vi "ChangeMotionParams.vi"(4 "newTrqGlobal":i32=4, 6 "newTrackingLimit":u32=100, 7 "newVelLimit":i32=2000, 8 "error in (no error)":errorcluster, 9 "newJrkLimit":i32=3, 10 "newAccelLimit":dbl format="%#_13g", 11 "Axis in":refnum<class "Axis.lvclass">) -> (0 "error out":errorcluster, 3 "Axis out":refnum<class "Axis.lvclass">)   [LabVIEW 2020, in "Axis.lvclass"]
uses:
  Axis.lvclass
  Axis.lvclass/Axis.ctl
  C:/Users/Jonathan/Documents/Clearpath SDK/CSharp Examples/CLRWrapper/x64/Debug/CLRWrapper.dll
  CSharp Examples/CLRWrapper/x64/Debug/CLRWrapper.dll
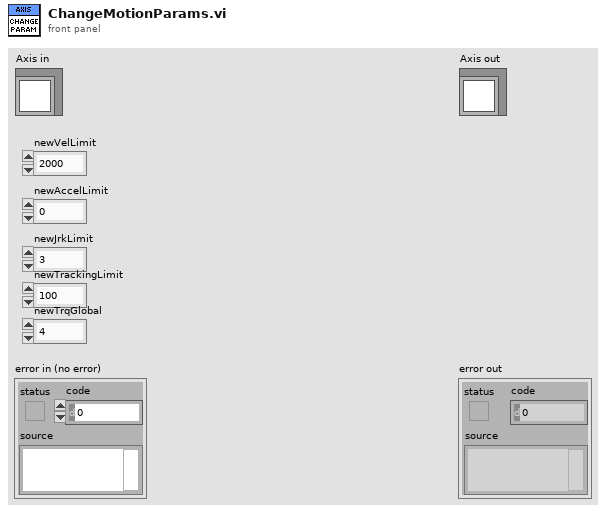
[diagram p1: front panel]
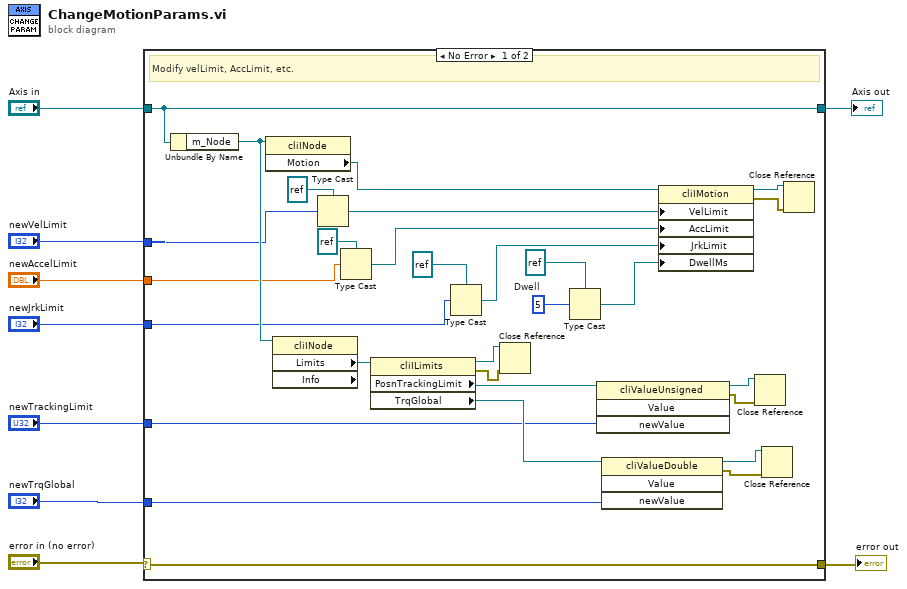
[diagram p0: block diagram]
diagram:
  n1 = case shown="No Error" "error in (no error)" {
    selector: "error in (no error)" -> [w38 w39]
    tunnel: [w38 w39] -> w4
    tunnel: "newVelLimit" -> [w36 _]
    tunnel: "newJrkLimit" -> [w35 _]
    tunnel: "Axis in" -> [w34 _]
    tunnel: [w34 _] -> w6
    tunnel: "newAccelLimit" -> [w20 _]
    tunnel: "newTrackingLimit" -> [w19 _]
    tunnel: "newTrqGlobal" -> [w18 _]
    frame No Error {
      w21 = 5  # Dwell
      # "Modify velLimit, AccLimit, etc."
      n2 = Unbundle By Name(w34) -> ("m_Node"=w37:refnum<k24>)
      n3 = property class="cliINode"(reference=w37) -> ("Motion"=w33:refnum<k24>)  [unwired: 1 in, 2 out]
      n4 = property class="cliINode" props=["Limits", "Info"](reference=w37) -> ("Limits"=w28:refnum<k24>)  [unwired: 1 in, 3 out]
      n5 = Type Cast(type=refnum<k24> refnum ("VelLimit"), x=w36) -> (*(type *) &x=w32:refnum<k24>)
      n6 = Type Cast(type=refnum<k24> refnum ("AccLimit"), x=w20) -> (*(type *) &x=w26:refnum<k24>)
      n7 = property class="cliILimits"(reference=w28) -> (reference out=w15:refnum<k24>, error out=w14:errorcluster, "PosnTrackingLimit"=w27:refnum<k24>, "TrqGlobal"=w24:refnum<k24>)  [unwired: 1 in]
      n8 = Type Cast(type=refnum<k24> refnum ("JrkLimit"), x=w35) -> (*(type *) &x=w25:refnum<k24>)
      n9 = Close Reference(reference=w15, error in (no error)=w14) -> ()  [unwired: 1 out]
      n10 = Type Cast(type=refnum<k24> refnum ("DwellMs"), x=w21) -> (*(type *) &x=w22:refnum<k24>)
      n11 = invoke class="cliValueUnsigned" method="Value"(reference=w27, "newValue"=w19) -> (reference out=w13:refnum<k24>, error out=w12:errorcluster)  [unwired: 2 in, 2 out]
      n12 = invoke class="cliValueDouble" method="Value"(reference=w24, "newValue"=w18) -> (reference out=w11:refnum<k24>, error out=w10:errorcluster)  [unwired: 2 in, 2 out]
      n13 = property class="cliIMotion"(reference=w33, "VelLimit"=w32, "AccLimit"=w26, "JrkLimit"=w25, "DwellMs"=w22) -> (reference out=w17:refnum<k24>, error out=w16:errorcluster)  [unwired: 1 in]
      n14 = Close Reference(reference=w13, error in (no error)=w12) -> ()  [unwired: 1 out]
      n15 = Close Reference(reference=w11, error in (no error)=w10) -> ()  [unwired: 1 out]
      n16 = Close Reference(reference=w17, error in (no error)=w16) -> ()  [unwired: 1 out]
    }
    frame Error {
    }
  }
  "error out" <- w4
  "Axis out" <- w6
